vi "Pre-Install Custom Action.vi"(10 "Variant":variant) -> (0 "error out":errorcluster)   [LabVIEW 2019]
uses:
  <vilib>/nisyscfg/Get Installed Components.vi
  <vilib>/nisyscfg/nisyscfg.lvlib
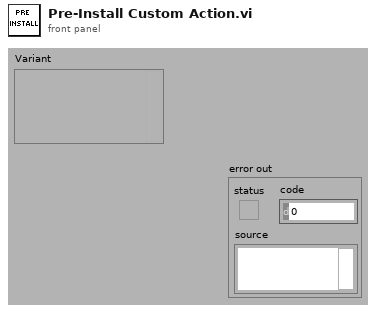
[diagram p1: front panel]
types:
  T1 = typedef "nisyscfg.lvlib/Software 1.2.ctl" = cluster{"title":string, "description":string, "ID":string, "version":string, "component type":T2}
  T2 = typedef "nisyscfg.lvlib/Component Type.ctl" = u32
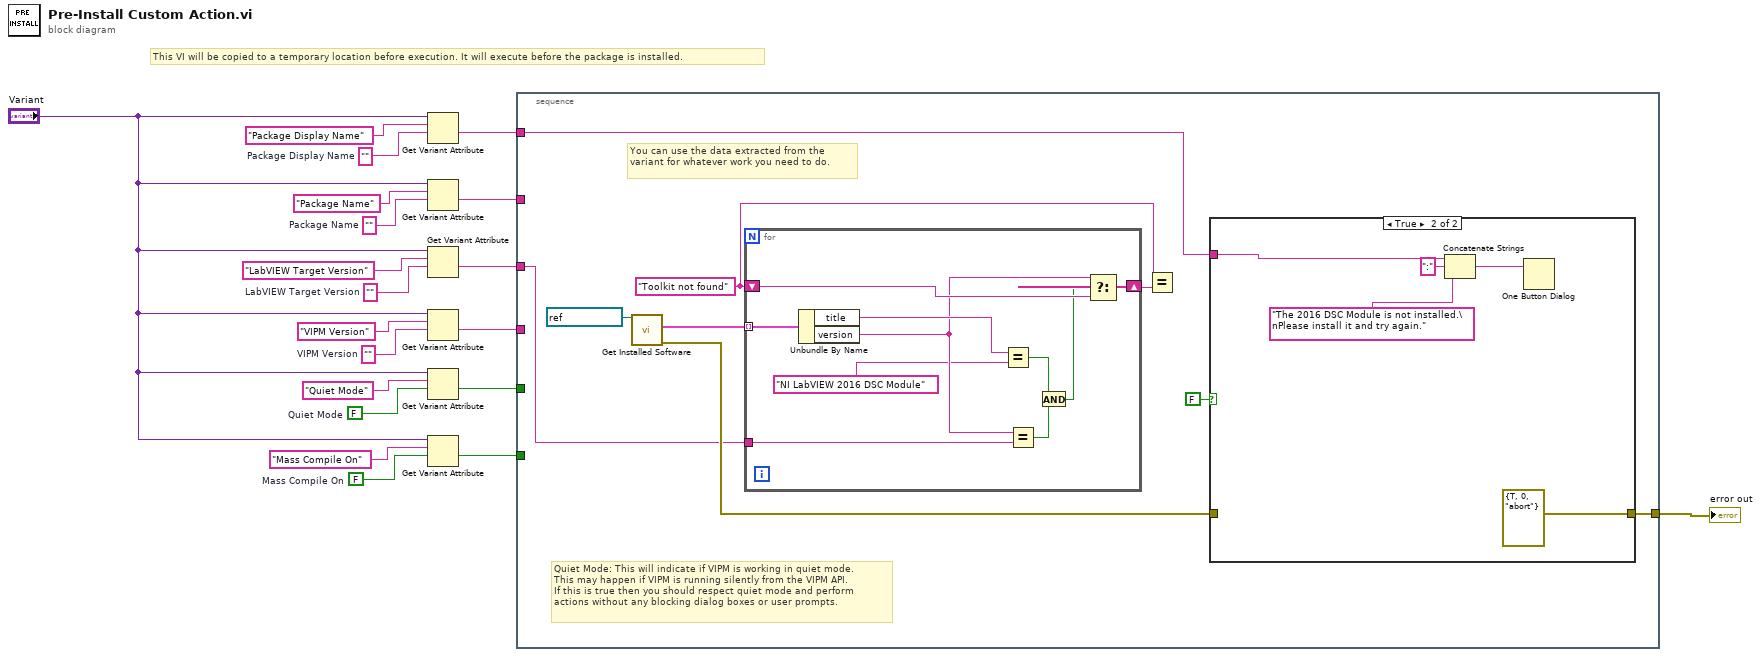
[diagram p0: block diagram]
diagram:
  w2 = FALSE  # Mass Compile On
  w4 = ""  # Package Display Name
  w11 = FALSE  # Quiet Mode
  w14 = ""  # VIPM Version
  w16 = ""  # LabVIEW Target Version
  w18 = ""  # Package Name
  # "This VI will be copied to a temporary location before execution. It will execute before the package is installed."
  n1 = Get Variant Attribute(Variant="Variant", name="Package Display Name", default value (empty Variant)=w4) -> (value=w10:string)  [unwired: 1 in, 3 out]
  n2 = Get Variant Attribute(Variant="Variant", name="Package Name", default value (empty Variant)=w18) -> (value=w9:string)  [unwired: 1 in, 3 out]
  n3 = Get Variant Attribute(Variant="Variant", name="LabVIEW Target Version", default value (empty Variant)=w16) -> (value=w8:string)  [unwired: 1 in, 3 out]
  n4 = Get Variant Attribute(Variant="Variant", name="VIPM Version", default value (empty Variant)=w14) -> (value=w7:string)  [unwired: 1 in, 3 out]
  n5 = Get Variant Attribute(Variant="Variant", name="Quiet Mode", default value (empty Variant)=w11) -> (value=w6:bool)  [unwired: 1 in, 3 out]
  n6 = Get Variant Attribute(Variant="Variant", name="Mass Compile On", default value (empty Variant)=w2) -> (value=w5:bool)  [unwired: 1 in, 3 out]
  n7 = stacked-sequence {
    tunnel: w10 -> [w22]
    tunnel: w9 -> [_]
    tunnel: w8 -> [w23]
    tunnel: w7 -> [_]
    tunnel: w6 -> [_]
    tunnel: w5 -> [_]
    tunnel: [w24] -> w1
    frame #0 {
      w28 = "Toolkit not found" ("version")
      # "Quiet Mode: This will indicate if VIPM is working in quiet mode.\nThis may happen if VIPM is running silently from the VIPM API.\nIf this is true then you should respect quiet mode and perform\nactions without any blocking dialog boxes or user prompts."
      # "You can use the data extracted from the variant for whatever work you need to do."
      n8 = call-poly <vilib>:"Get Installed Software.vi"("Session in"=refnum<k21> "localhost") -> ("error out"=w29:errorcluster, "Software Components"=w26:T1[])  [unwired: 8 in, 1 out]
      n9 = for {
        tunnel: w26 -> [w45] mode=indexing
        shift-right: [w43] -> w25
        shift-left: w28 -> [w42]
        tunnel: w23 -> [w37]
        n10 = Unbundle By Name(w45) -> ("title"=w44:string, "version"=w41:string)
        n11 = Equal?(x=w44, y="NI LabVIEW 2016 DSC Module" ("regular expression")) -> (x = y?=w40:bool)
        n12 = Equal?(x=w41, y=w37) -> (x = y?=w39:bool)
        n13 = And(x=w40, y=w39) -> (x .and. y?=w38:bool)
        n14 = Select(t=w41, s=w38, f=w42) -> (s? t:f=w43:string)
      }
      n15 = Equal?(x=w28, y=w25) -> ()  [unwired: 1 out]
      n16 = case shown="True" FALSE {
        tunnel: [w30 errorcluster {"status"=TRUE, "code"=0, "source"="abort"} ("error out")] -> w24
        tunnel: w29 -> [w30 _]
        tunnel: w22 -> [_ w33]
        frame False {
        }
        frame True {
          n17 = Concatenate Strings(w33, ":" ("string"), "The 2016 DSC Module is not installed.\nPlease install it and try again." ("message")) -> (w31:string)
          n18 = One Button Dialog(message=w31) -> ()  [unwired: 1 in, 1 out]
        }
      }
    }
  }
  "error out" <- w1
